vi "Actor Core.vi"(8 "error in":errorcluster, 11 "RP I-V in":refnum<class "RP I-V.lvclass">) -> (0 "error out":errorcluster, 3 "Actor out":refnum<class "Actor.lvclass">)   [LabVIEW 2018, in "RP I-V.lvclass"]
doc: "(<B>Filename</B>: Actor Framework.lvlib:Actor.lvclass:Actor Core.vi)\n\nReceives messages to the actor, reacts to them, and initiates any error handling that may shut the actor down.\n\nDescendant classes may override this VI to append parallel tasks for the actor to complete while it handles messages. Overrides use the Call Parent Method node."
uses:
  RP I-V.lvclass
  <vilib>/ActorFramework/Actor/Actor.lvclass
  NHMFL_Core/Libraries/Red Pitaya/RP Core/Rep Pitaya I-V driver/RP I-V Configuration.ctl
  NHMFL_Core/Libraries/Red Pitaya/Waform generation/I-V parameters.ctl
  RP I-V.lvclass/RP I-V.ctl
  Pulse Recorders/Pulse Recorder/Pulse Recorder.lvclass
panel:
  out "Output Waveform":i16[](graph)
  out "Armed":bool
  out "Name":string
  in  "Configuration":T1={"I-V parameters"={"Start magnitude"=0.001, "Magnitude increment"=0.001, "End magnitude"=0.01, "Ramp length"=32, "Top  length"=480, "Threshold "=0.0001, "Processing delay"=22, "Valhalla range"=0.01, "Interpolation"=64, "Stop after"=1, "Detector window"=480}, "Ranges"=[1.0, 1.0], "Pre-trigger duration"=0.001, "Post-trigger duration"=0.1, "Output delay"=0.001} {"Output delay" format="%#_6ps"; "Post-trigger duration" format="%#_6ps"; "Pre-trigger duration" format="%#_6ps"; "Ranges" format="%#_6pV"; "I-V parameters"."Detector window" format="%dpts"; "I-V parameters"."Stop after" format="%d sweep(s)"; "I-V parameters"."Valhalla range" format="%#_6pA"; "I-V parameters"."Processing delay" format="%dpts"; "I-V parameters"."Threshold" format="%#_6pV"; "I-V parameters"."Top  length" format="%dpts"; "I-V parameters"."Ramp length" format="%dpts"; "I-V parameters"."End magnitude" format="%#_6pA"; "I-V parameters"."Magnitude increment" format="%#_6pA"; "I-V parameters"."Start magnitude" format="%#_6pA"}
  # "Waveform parameters"
  # "Detector parameters"
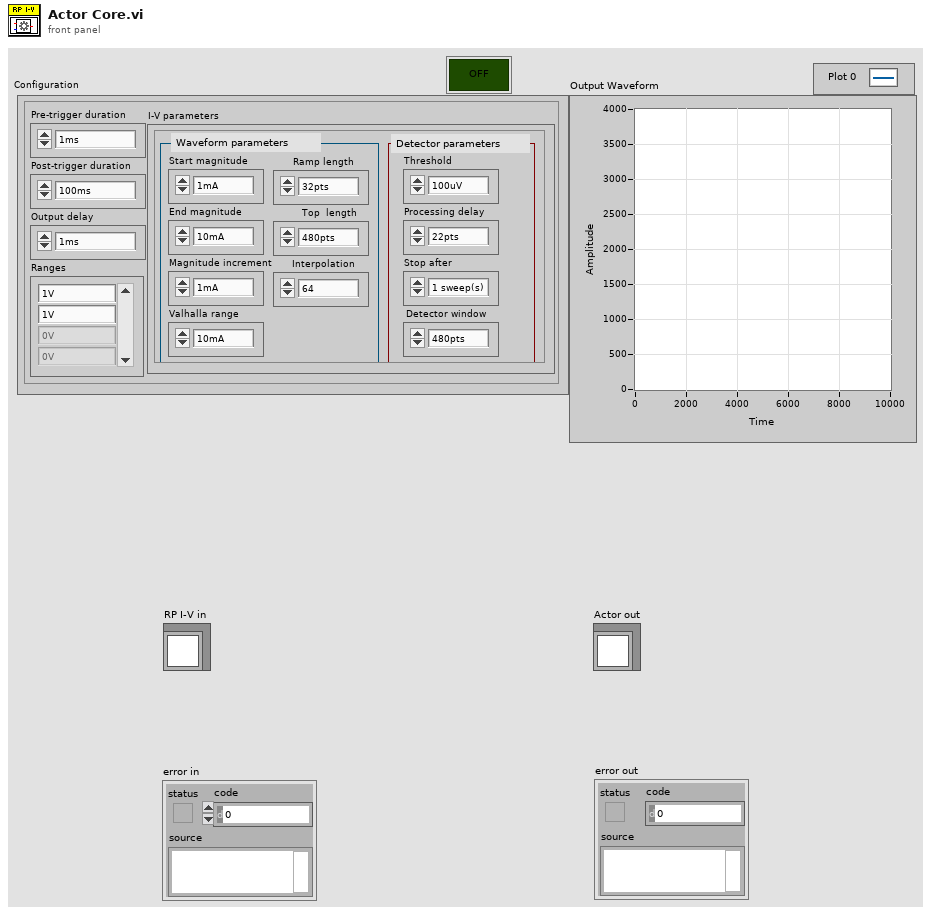
[diagram p1: front panel]
types:
  T1 = typedef "RP I-V Configuration.ctl" = cluster{"I-V parameters":T2, "Ranges":dbl[], "Pre-trigger duration":dbl, "Post-trigger duration":dbl, "Output delay":dbl}
  T2 = typedef "I-V parameters.ctl" = cluster{"Start magnitude":dbl, "Magnitude increment":dbl, "End magnitude":dbl, "Ramp length":i32, "Top  length":i32, "Threshold ":dbl, "Processing delay":u16, "Valhalla range":dbl, "Interpolation":i32, "Stop after":u16, "Detector window":i32}
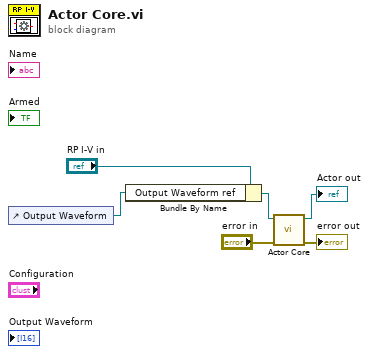
[diagram p0: block diagram]
diagram:
  n1 = control-ref of="Output Waveform"() -> (w1:refnum<vi>)
  n2 = Bundle By Name(cluster="RP I-V in", "Output Waveform ref"=w1) -> (w2:refnum<class "RP I-V.lvclass">)
  n3 = call-parent "Actor Core.vi"("error in"="error in", "Pulse Recorder in"=w2) -> ("error out"=→"error out":errorcluster, "Actor out"=→"Actor out":refnum<class "Actor.lvclass">)  [unwired: 8 in]
